vi "SRC_sensor_vi.vi"(11 "VISA Resource Name":refnum<visa-resource-name>="GPIB0::9::INSTR") -> (0 "Temperature":dbl, 3 "VISA Resource Name Out":refnum<visa-resource-name>)   [LabVIEW 2017]
uses:
  <instrlib>/Agilent 34970/Agilent 34970.lvlib
panel:
  out "Current measure":dbl[](array[numeric]) format="%.7f"
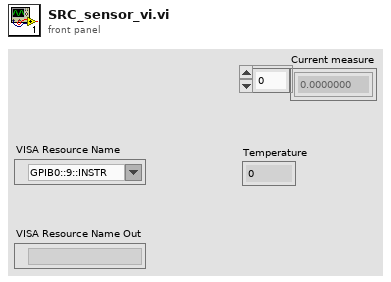
[diagram p1: front panel]
types:
  T1 = enum16{"4 1/2", "5 1/2", "6 1/2", "Least", "Highest", "Default"}
  T2 = enum16{"10 mA", "100 mA", "1 A", "Auto", "Minimum", "Maximum"}
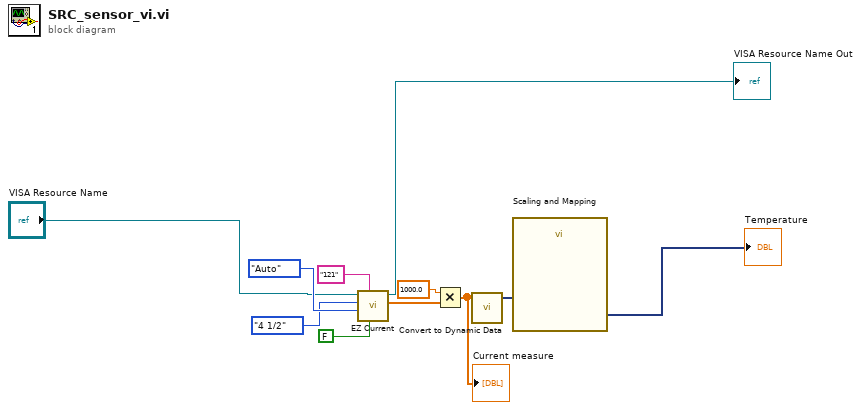
[diagram p0: block diagram]
diagram:
  n1 = call <instrlib>:"EZ Current.vi"("DC/AC (F:DC)"=FALSE, "Scan List (empty)"="121" ("Channel List"), "Range (3:Auto)"=T2."Auto", "Resolution (3:Least)"=T1."4 1/2", "VISA Resource Name"="VISA Resource Name") -> ("Output Array"=w8:dbl[], "VISA Resource Name Out"=→"VISA Resource Name Out":refnum<visa-resource-name>)  [unwired: 4 in, 1 out]
  n2 = Multiply(x=1000.0, y=w8) -> (x*y=w7:dbl[])
  "Current measure" <- w7
  n3 = call "Convert to Dynamic Data"("Array"=w7) -> ("Dynamic Data Type"=w9:dynamicdata)  [unwired: 3 in]
  n4 = call "Scaling and Mapping"("Signals"=w9) -> ("Scaled Signals"=→"Temperature":dynamicdata)  [unwired: 9 in, 1 out]
